vi "buffer calling (1d array).vi"() -> ()   [LabVIEW 2021]
panel:
  out "Time (ms)":i32
  out "buffer out":dbl[](array[numeric]) format="%.2f"
  in  "Iteration":u16
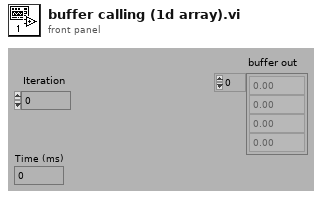
[diagram p1: front panel]
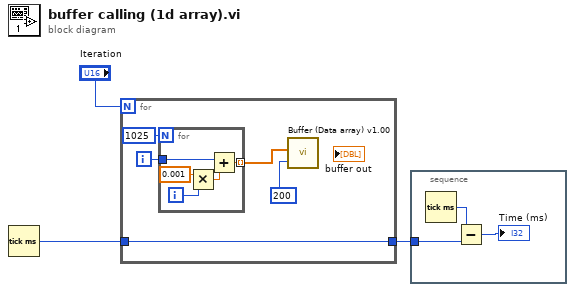
[diagram p0: block diagram]
diagram:
  n1 = Tick Count (ms)() -> (millisecond timer value=w2:u32)
  n2 = for {
    N: "Iteration" -> [_]
    tunnel: [w4] -> w1
    tunnel: w2 -> [w4]
    i -> [w6]
    n3 = for {
      N: 1025 -> [_]
      tunnel: w6 -> [w10]
      tunnel: [w9] -> w5 mode=indexing
      i -> [w12]
      n4 = Multiply(x=0.001, y=w12) -> (x*y=w11:dbl)
      n5 = Add(x=w10, y=w11) -> (x+y=w9:dbl)
    }
    n6 = call "Buffer (Data array) v1.00.vi"("Read#"=200 ("Max Buffer Size"), "Y Data In"=w5) -> ()  [unwired: 6 in, 4 out]
  }
  n7 = stacked-sequence {
    tunnel: w1 -> [w15]
    frame #0 {
      n8 = Tick Count (ms)() -> (millisecond timer value=w14:u32)
      n9 = Subtract(x=w14, y=w15) -> (x-y=→"Time (ms)":u32)
    }
  }
